vi "SerialReadSpeedTest.vi"() -> ()   [LabVIEW 2013]
uses:
  <vilib>/Instr/_visa.llb/VISA Configure Serial Port (Instr).vi
panel:
  out "XY Graph":cluster{i32[], "unsigned byte array":u8[]}(graph)
  out "unsigned byte array 2":u8[][](array[numeric])
  out "unsigned byte array":u8[](array[numeric])
  out "cell":u8[](array[numeric])
  out "output_int16":i32[](array[numeric])
  in  "baud rate":u32=9600
  out "time dt(ms)":dbl
  in  "t2":dbl
  in  "t1":dbl
  in  "stop":bool
  in  "serial_port":refnum<visa-resource-name> caption="Porta Serial"
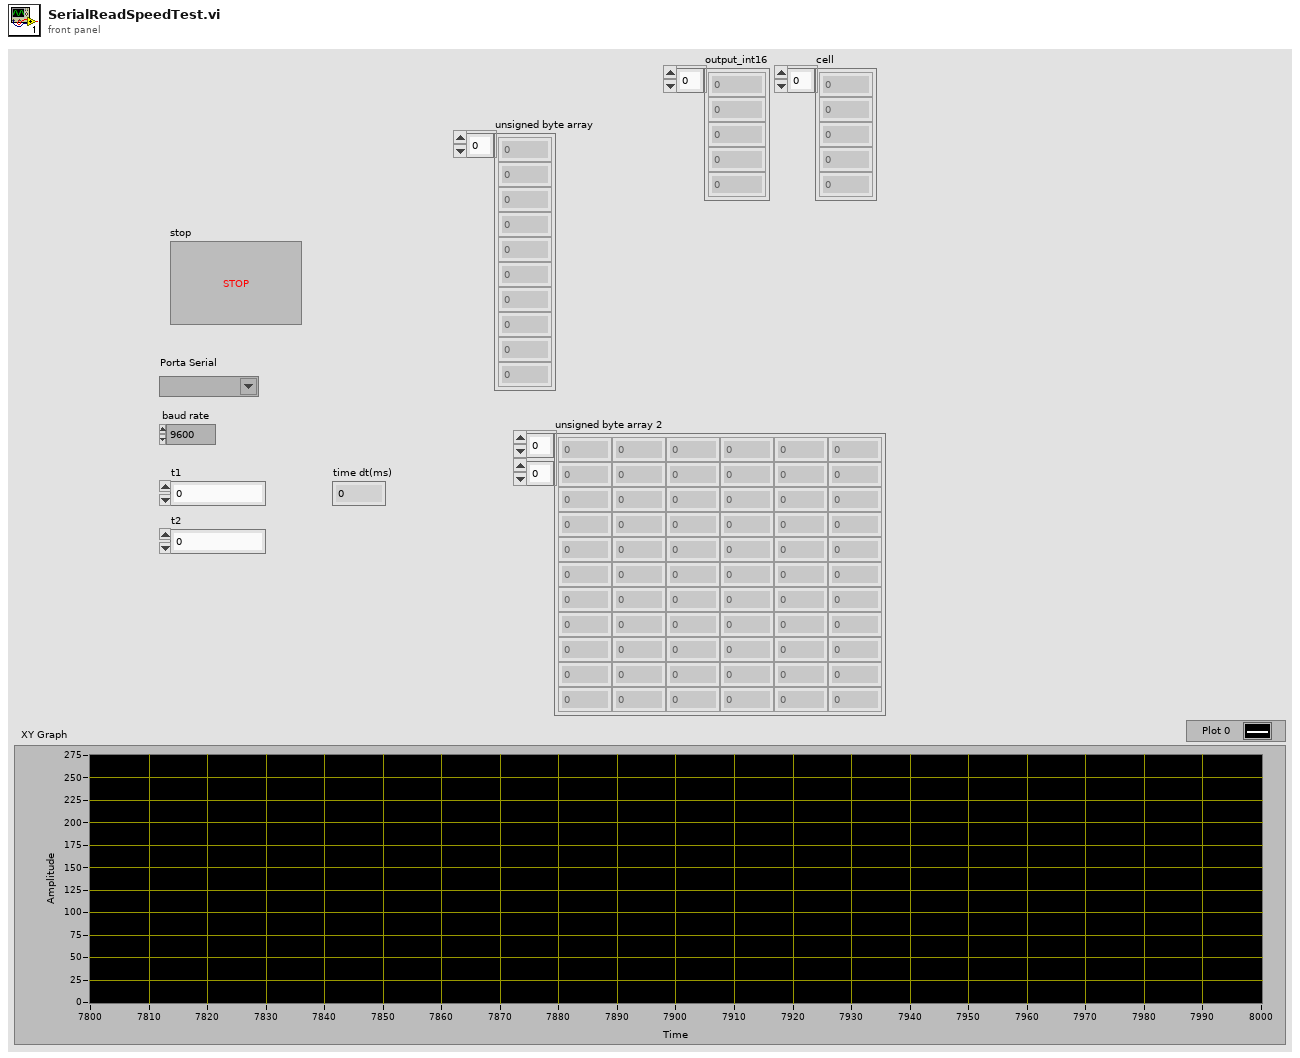
[diagram p1: front panel]
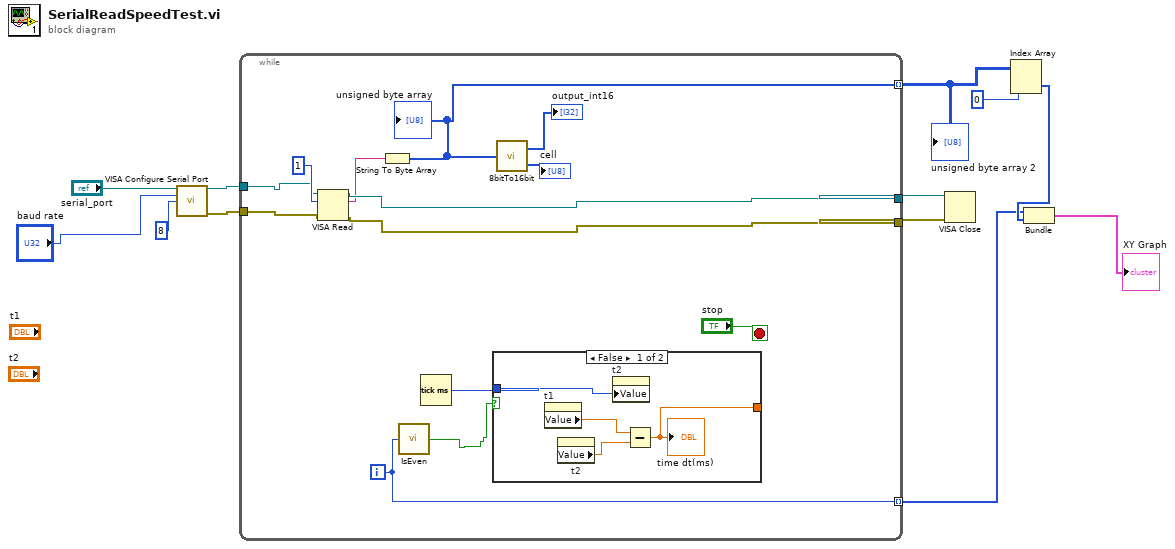
[diagram p0: block diagram]
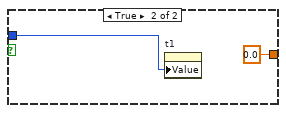
[diagram p2: hidden frame]
diagram:
  n1 = call-poly "VISA Configure Serial Port"("VISA resource name"="serial_port", "baud rate (9600)"="baud rate", "data bits (8)"=u16 8) -> ("VISA resource name out"=w10:refnum<visa-resource-name>, "error out"=w9:errorcluster)  [unwired: 11 in]
  n2 = while {
    tunnel: w10 -> [w20]
    tunnel: w9 -> [w21]
    tunnel: [w18] -> w8
    tunnel: [w19] -> w7
    tunnel: [w14] -> w2 mode=indexing
    tunnel: [w13] -> w5 mode=indexing
    i -> [w14]
    stop <- "stop" stop-if-true
    n3 = VISA Read(VISA resource name=w20, byte count=1, error in (no error)=w21) -> (VISA resource name out=w19:refnum<visa-resource-name>, read buffer=w17:string, error out=w18:errorcluster)  [unwired: 1 out]
    n4 = String To Byte Array(string=w17) -> (unsigned byte array=w13:u8[])
    "unsigned byte array" <- w13
    n5 = call "IsEven.vi"("Numeric"=w14) -> ("Boolean"=w23:bool)
    n6 = Tick Count (ms)() -> (millisecond timer value=w24:u32)
    n7 = case shown="False" w23 {
      tunnel: w24 -> [w29 w31]
      tunnel: [w26 0.0] -> _
      frame False {
        n8 = property on="t1" class="DigNum (strict)"() -> ("Value"=w28:dbl)  [unwired: 2 in, 2 out]
        n9 = property on="t2" class="DigNum (strict)"() -> ("Value"=w27:dbl)  [unwired: 2 in, 2 out]
        n10 = property on="t2" class="DigNum (strict)"("Value"=w29) -> ()  [unwired: 2 in, 2 out]
        n11 = Subtract(x=w28, y=w27) -> (x-y=w26:dbl)
        "time dt(ms)" <- w26
      }
      frame True {
        n12 = property on="t1" class="DigNum (strict)"("Value"=w31) -> ()  [unwired: 2 in, 2 out]
      }
    }
    n13 = call "8bitTo16bit.vi"("input_byte"=w13) -> ("output_int16"=→"output_int16":i32[], "cell"=→"cell":u8[])
  }
  "unsigned byte array 2" <- w5
  n14 = VISA Close(VISA resource name=w7, error in (no error)=w8) -> ()  [unwired: 1 out]
  n15 = Index Array(array=w5, index (col)=0 ("disabled index (col)")) -> (element=w3:u8[])  [unwired: 1 in]
  n16 = Bundle(w2, "unsigned byte array"=w3) -> (→"XY Graph":cluster{i32[], "unsigned byte array":u8[]})  [unwired: 1 in]
